vi "Teleop.vi"(10 "Match Info":T1={"Autonomous Elapsed Seconds"=0.0, "TeleOp Elapsed Seconds"=0.0, "Disabled Elapsed Seconds"=0.0, "Visited Autonomous"=FALSE, "Visited TeleOp"=FALSE, "Visited Disabled"=FALSE, "Autonomous Settings"={"Autonomous Style"=enum."Independent", "VI Refnum"=refnum}}, 11 "Call Context":T2) -> ()   [LabVIEW 2014]
doc: "This VI is called for each TeleOp packet received from the DS where the robot is not disabled. It is often used to read from the joysticks and update I/O or to update setpoints for timed control loops. It should complete and return within 20 milliseconds or it may miss DS packets."
uses:
  <vilib>/Rock Robotics/WPI/DriverStation/WPI_DriverStationDerivedRobotMode.ctl
  <vilib>/Rock Robotics/WPI/DriverStation/WPI_DriverStationMatch Info.ctl
  <vilib>/Rock Robotics/WPI/RobotDrive/WPI_RobotDriveGetSetRefNum.vi
  <vilib>/Rock Robotics/WPI/Joystick/WPI_JoystickGetSetRefNum.vi
  <vilib>/Rock Robotics/Network Tables/SD Write Boolean Array.vi
  <vilib>/Rock Robotics/Network Tables/SD Write Numeric Array.vi
  <vilib>/Rock Robotics/Network Tables/SD Write Boolean.vi
  <vilib>/Rock Robotics/WPI/RobotDrive/WPI_RobotDriveMecanumDrive_Cartesian.vi
  <vilib>/addons/control/pid/pid.llb/PID Advanced (DBL).vi
  <vilib>/addons/control/pid/NI_PID_pid.lvlib
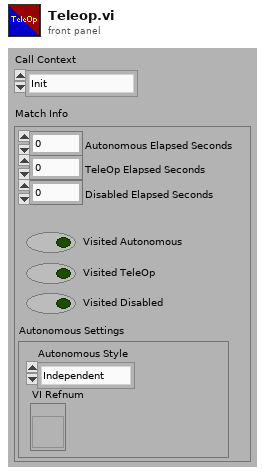
[diagram p1: front panel]
types:
  T1 = typedef "WPI_DriverStationMatch Info.ctl" = cluster{"Autonomous Elapsed Seconds":dbl, "TeleOp Elapsed Seconds":dbl, "Disabled Elapsed Seconds":dbl, "Visited Autonomous":bool, "Visited TeleOp":bool, "Visited Disabled":bool, "Autonomous Settings":cluster{"Autonomous Style":enum16{"Iterative", "Independent"}, "VI Refnum":refnum<vi>}}
  T2 = typedef "WPI_DriverStationDerivedRobotMode.ctl" = enum16{"Init", "Execute", "Stop"}
  T3 = cluster{"proportional gain (Kc)":dbl, "integral time (Ti, min)":dbl, "derivative time (Td, min)":dbl}
  T4 = typedef "WPI_JoystickDevRef.ctl" = cluster{"Device":T5}
  T5 = typedef "WPI_JoystickDeviceEnum.ctl" = enum16{"USB 0", "USB 1", "USB 2", "USB 3", "USB 4", "USB 5"}
  T6 = typedef "WPI_RobotDriveDevRef.ctl" = cluster{"DevStatus":errorcluster, "Motors[]":T7[], "Square Inputs":bool, "Max Output":dbl}
  T7 = typedef "WPI_MotorControlDeviceRef.ctl" = cluster{"DeviceStatus":errorcluster, "Type":T8, "PWM":cluster{"Controller":T9, "PWM Channel":T10, "DeadBand":T11}, "CAN":cluster{"Device Number":u8, "Control Mode":T12, "Semaphore":T13, "Max Vout":dbl, "TalonSRX Control Mode":T14}, "Invert":bool, "TransformRef":T15, "InvTransformRef":T15}
  T8 = typedef "WPI_MotorControlType.ctl" = enum16{"PWM", "CAN", "CANTalonSRX"}
  T9 = typedef "FPGA_TypedefDigitalModule.ctl" = enum16{"Controller 1"}
  T10 = typedef "FPGA_DIOPWMChannel.ctl" = enum8{"PWM 0", "PWM 1", "PWM 2", "PWM 3", "PWM 4", "PWM 5", "PWM 6", "PWM 7", "PWM 8", "PWM 9", "PWM MXP 0", "PWM MXP 1", "PWM MXP 2", "PWM MXP 3", "PWM MXP 4", "PWM MXP 5", "PWM MXP 6", "PWM MXP 7", "PWM MXP 8", "PWM MXP 9", "Invalid"}
  T11 = typedef "WPI_PWMDeadband.ctl" = cluster{"Name":string, "maxPositivePwm":i32, "minPositivePwm":i32, "centerPwm":i32, "maxNegativePwm":i32, "minNegativePwm":i32, "angularRange":u16}
  T12 = typedef "WPI_CANJaguar_ControlMode.ctl" = enum8{"Percent VBus", "Current", "Speed", "Position", "Voltage"}
  T13 = typedef "Semaphore RefNum" = refnum<k1>
  T14 = typedef "WPI_CANTalonSRX_APIControlMode.ctl" = enum8{"Percent VBus", "Speed", "Position", "Slave", "Unchanged / Invalid"}
  T15 = typedef "WPI_PWMTransform_ConPane.ctl" = refnum<vi>
  T16 = cluster{"Axes[0]":dbl, "Axes[1]":dbl, "Axes[2]":dbl, "Axes[3]":dbl, "Axes[4]":dbl, "Axes[5]":dbl, "Axes[6]":dbl, "Axes[7]":dbl, "Axes[8]":dbl}
  T17 = typedef "WPI_EncoderDevRef.ctl" = cluster{"DevStatus":errorcluster, "EncoderIndex":T18, "CounterIndex":T19, "DistancePerCount":dbl, "Decoding Type":T20}
  T18 = typedef "FPGA_EncoderIdx.ctl" = enum8{"Enc 0", "Enc 1", "Enc 2", "Enc 3", "Enc 4", "Enc 5", "Enc 6", "Enc 7", "Invalid"}
  T19 = typedef "FPGA_CounterCtrSystemIndex.ctl" = enum8{"Ctr 0", "Ctr 1", "Ctr 2", "Ctr 3", "Ctr 4", "Ctr 5", "Ctr 6", "Ctr 7", "Invalid"}
  T20 = typedef "WPI_EncoderType.ctl" = enum16{"1x", "2x", "4x"}
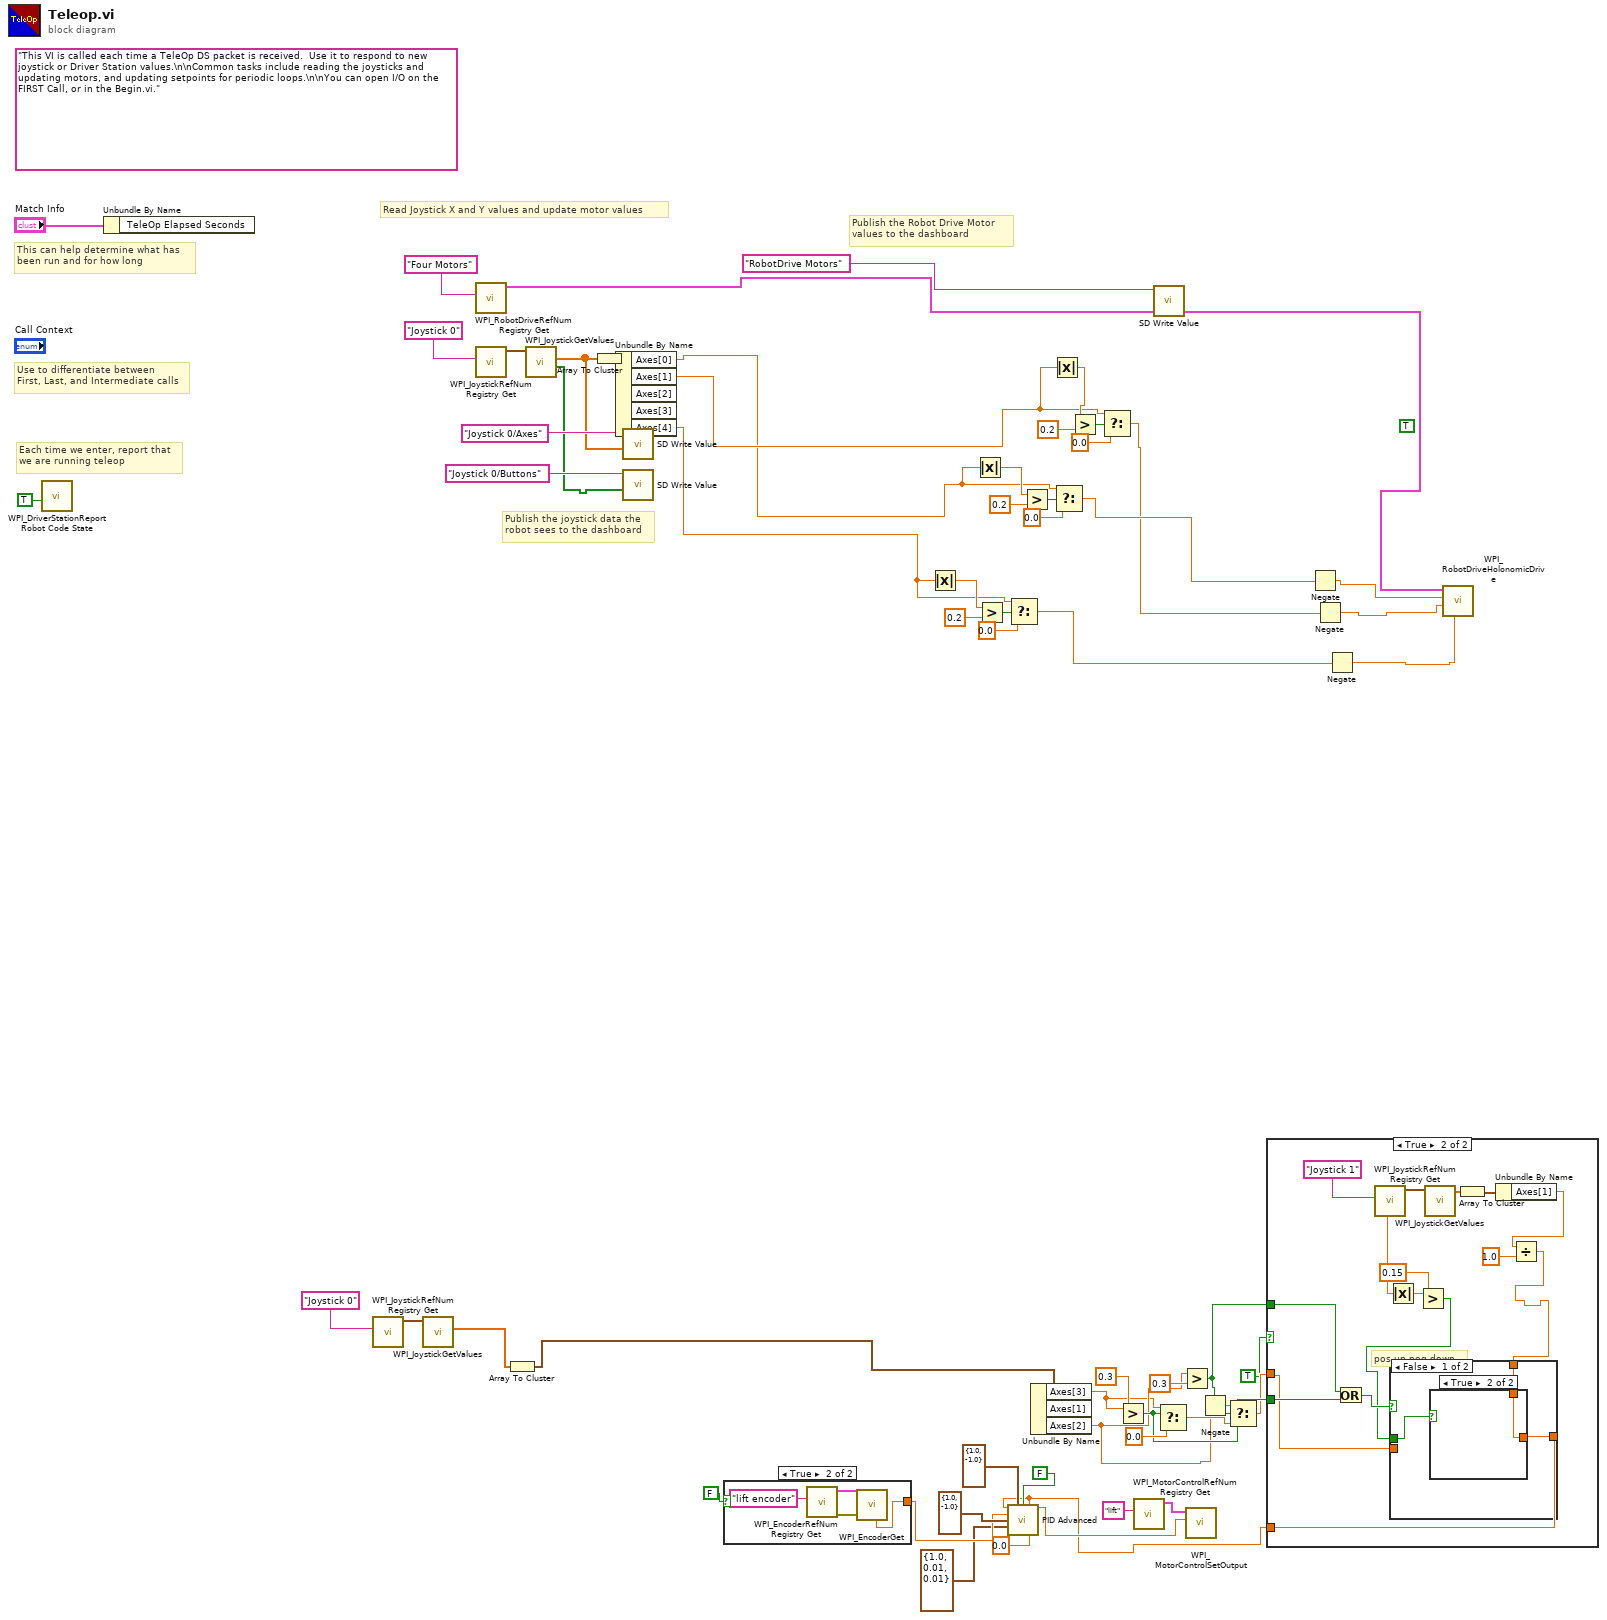
[diagram p0: block diagram]
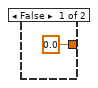
[diagram p4: hidden frame]
diagram:
  (unwired) TRUE ("practice bot")
  (unwired) "This VI is called each time a TeleOp DS packet is received.  Use it to respond to new joystick or Driver Station values.\n\nCommon tasks include reading the joysticks and updating motors, and updating setpoints for periodic loops.\n\nYou can open I/O on the FIRST Call, or in the Begin.vi."
  # "Publish the Robot Drive Motor\nvalues to the dashboard"
  # "Publish the joystick data the\nrobot sees to the dashboard"
  # "Each time we enter, report that\nwe are running teleop"
  # "Use to differentiate between\nFirst, Last, and Intermediate calls"
  # "This can help determine what has\nbeen run and for how long"
  # "Read Joystick X and Y values and update motor values"
  n1 = call <vilib>:"WPI_DriverStationReport Robot Code State.vi"("TeleOp"=TRUE ("Autonomous")) -> ()  [unwired: 10 in, 1 out]
  n2 = Unbundle By Name("Match Info") -> ()  [unwired: 1 out]
  n3 = call <vilib>:"WPI_JoystickRefNum Registry Get.vi"("refnum name"="Joystick 0") -> ("JoystickDevRef"=w40:T4)  [unwired: 1 in, 9 out]
  n4 = call <vilib>:"WPI_JoystickGetValues.vi"("JoystickDevRef"=w40) -> ("Axes"=w39:dbl[])  [unwired: 6 in, 4 out]
  n5 = call <vilib>:"WPI_RobotDriveRefNum Registry Get.vi"("refnum name"="Four Motors") -> ("RobotDriveDevRef"=w5:T6)  [unwired: 1 in, 9 out]
  n6 = call <vilib>:"WPI_JoystickRefNum Registry Get.vi"("refnum name"="Joystick 0") -> ("JoystickDevRef"=w56:T4)  [unwired: 1 in, 9 out]
  n7 = Array To Cluster(array=w39) -> (cluster=w38:T16)
  n8 = call <vilib>:"WPI_JoystickGetValues.vi"("JoystickDevRef"=w56) -> ("Buttons"=w42:bool[], "Axes"=w51:dbl[])  [unwired: 6 in, 3 out]
  n9 = Array To Cluster(array=w51) -> (cluster=w50:T16)
  n10 = Unbundle By Name(w50) -> ("Axes[0]"=w23:dbl, "Axes[1]"=w25:dbl, "Axes[4]"=w14:dbl)  [unwired: 2 out]
  n11 = call-poly <vilib>:"SD Write Value.vi"("Numeric Array"=w51, "Name"="Joystick 0/Axes") -> ()  [unwired: 8 in, 2 out]
  n12 = call-poly <vilib>:"SD Write Value.vi"("Boolean Array"=w42, "Name"="Joystick 0/Buttons") -> ()  [unwired: 8 in, 2 out]
  n13 = case shown="True" FALSE {
    tunnel: [_ w60] -> w46
    frame False {
    }
    frame True {
      n14 = call <vilib>:"WPI_EncoderRefNum Registry Get.vi"("refnum name"="lift encoder") -> ("error out"=w63:errorcluster, "EncoderDevRef"=w62:T17)  [unwired: 9 in]
      n15 = call <vilib>:"WPI_EncoderGet.vi"("error in (no error)"=w63, "EncoderDevRef"=w62) -> ("Rate"=w60:dbl)  [unwired: 4 in, 5 out]
    }
  }
  n16 = Absolute Value(x=w14) -> (abs(x)=w15:dbl)
  n17 = Absolute Value(x=w23) -> (abs(x)=w24:dbl)
  n18 = Greater?(x=w15, y=0.2) -> (0:w18:bool)
  n19 = Select(t=w14, s=w18, f=0.0) -> (s? t:f=w8:dbl)
  n20 = Greater?(x=w24, y=0.2) -> (0:w30:bool)
  n21 = Unbundle By Name(w38) -> ("Axes[3]"=w10:dbl, "Axes[2]"=w11:dbl)  [unwired: 1 out]
  n22 = Absolute Value(x=w25) -> (abs(x)=w26:dbl)
  n23 = Select(t=w23, s=w30, f=0.0) -> (s? t:f=w7:dbl)
  n24 = Greater?(x=w26, y=0.2) -> (0:w32:bool)
  n25 = Select(t=w25, s=w32, f=0.0) -> (s? t:f=w6:dbl)
  n26 = Greater?(x=w10, y=0.3) -> (0:w22:bool)
  n27 = call <vilib>:"WPI_MotorControlRefNum Registry Get.vi"("refnum name"="lift") -> ("MotorControlDevRef"=w43:T7)  [unwired: 9 in, 1 out]
  n28 = call-poly <vilib>:"SD Write Value.vi"("Name"="RobotDrive Motors") -> ()  [unwired: 9 in, 2 out]
  n29 = Select(t=w10, s=w22, f=0.0) -> (s? t:f=w21:dbl)
  n30 = Greater?(x=w11, y=0.3) -> (0:w20:bool)
  n31 = Negate(x=w11) -> (-x=w12:dbl)
  n32 = Select(t=w12, s=w20, f=w21) -> (s? t:f=w19:dbl)
  n33 = case shown="True" TRUE {
    tunnel: w22 -> [_ w74]
    tunnel: [w64 w73] -> w1
    tunnel: w20 -> [_ w69]
    tunnel: w19 -> [w64 w68]
    frame False {
    }
    frame True {
      # "pos up neg down"
      n34 = Or(x=w69, y=w74) -> (x .or. y?=w75:bool)
      n35 = call <vilib>:"WPI_JoystickRefNum Registry Get.vi"("refnum name"="Joystick 1") -> ("JoystickDevRef"=w78:T4)  [unwired: 1 in, 9 out]
      n36 = call <vilib>:"WPI_JoystickGetValues.vi"("JoystickDevRef"=w78) -> ("Axes"=w77:dbl[])  [unwired: 6 in, 4 out]
      n37 = Array To Cluster(array=w77) -> (cluster=w76:T16)
      n38 = Unbundle By Name(w76) -> ("Axes[1]"=w67:dbl)
      n39 = Absolute Value(x=w67) -> (abs(x)=w72:dbl)
      n40 = Greater?(x=w72, y=0.15) -> (0:w70:bool)
      n41 = Divide(x=w67, y=1.0) -> (x/y=w65:dbl)
      n42 = case shown="False" w75 {
        tunnel: w70 -> [w82 _]
        tunnel: [w81 w85] -> w73
        tunnel: w68 -> [_ w85]
        tunnel: w65 -> [w80 _]
        frame False {
          n43 = case shown="True" w82 {
            tunnel: [0.0 w84] -> w81
            tunnel: w80 -> [_ w84]
            frame False {
            }
            frame True {
            }
          }
        }
        frame True {
        }
      }
    }
  }
  n44 = call-poly <vilib>:"PID Advanced.vi"("setpoint"=w1, "output range"=cluster{"output high":dbl, "output low":dbl} {"output high"=1.0, "output low"=-1.0}, "auto? (T)"=FALSE, "manual control"=w1, "process variable"=w46, "setpoint range"=cluster{"setpoint high":dbl, "setpoint low":dbl} {"setpoint high"=1.0, "setpoint low"=-1.0}, "PID gains"=T3 {"proportional gain (Kc)"=1.0, "integral time (Ti, min)"=0.01, "derivative time (Td, min)"=0.01}, "linearity"=0.0) -> ("output"=w33:dbl)  [unwired: 6 in, 1 out]
  n45 = call <vilib>:"WPI_MotorControlSetOutput.vi"("Output"=w33, "MotorControlDevRef"=w43) -> ()  [unwired: 7 in, 3 out]
  n46 = Negate(x=w7) -> (-x=w3:dbl)
  n47 = Negate(x=w6) -> (-x=w4:dbl)
  n48 = Negate(x=w8) -> (-x=w2:dbl)
  n49 = call-poly <vilib>:"WPI_RobotDriveHolonomicDrive.vi"("Rotation"=w2, "Y"=w4, "X"=w3, "RobotDriveDevRef"=w5) -> ()  [unwired: 5 in, 3 out]
